vi "Validate Remote Session.vi"(0 "Session in":refnum<class "Remote Connection Session.lvclass">, 11 "error in":errorcluster) -> (4 "Session out":refnum<class "Remote Connection Session.lvclass">, 15 "error out":errorcluster)   [LabVIEW 2012, in "REx.lvlib" / "Remote Connection Session.lvclass"]
uses:
  Remote Connection Session.lvclass
  Remote Connection Session.lvclass/Remote Connection Session.ctl
  Local Listener Session/Obtain Session.vi
  Local Listener Session/Release Session.vi
  Local Listener Session/Local Listener Session.lvclass
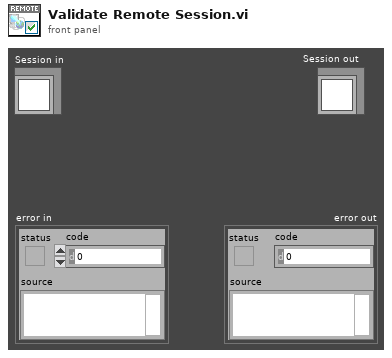
[diagram p1: front panel]
types:
  T1 = typedef "REx.lvlib/Local Listener Session.lvclass/Session Handle.ctl" = refnum<data-value>
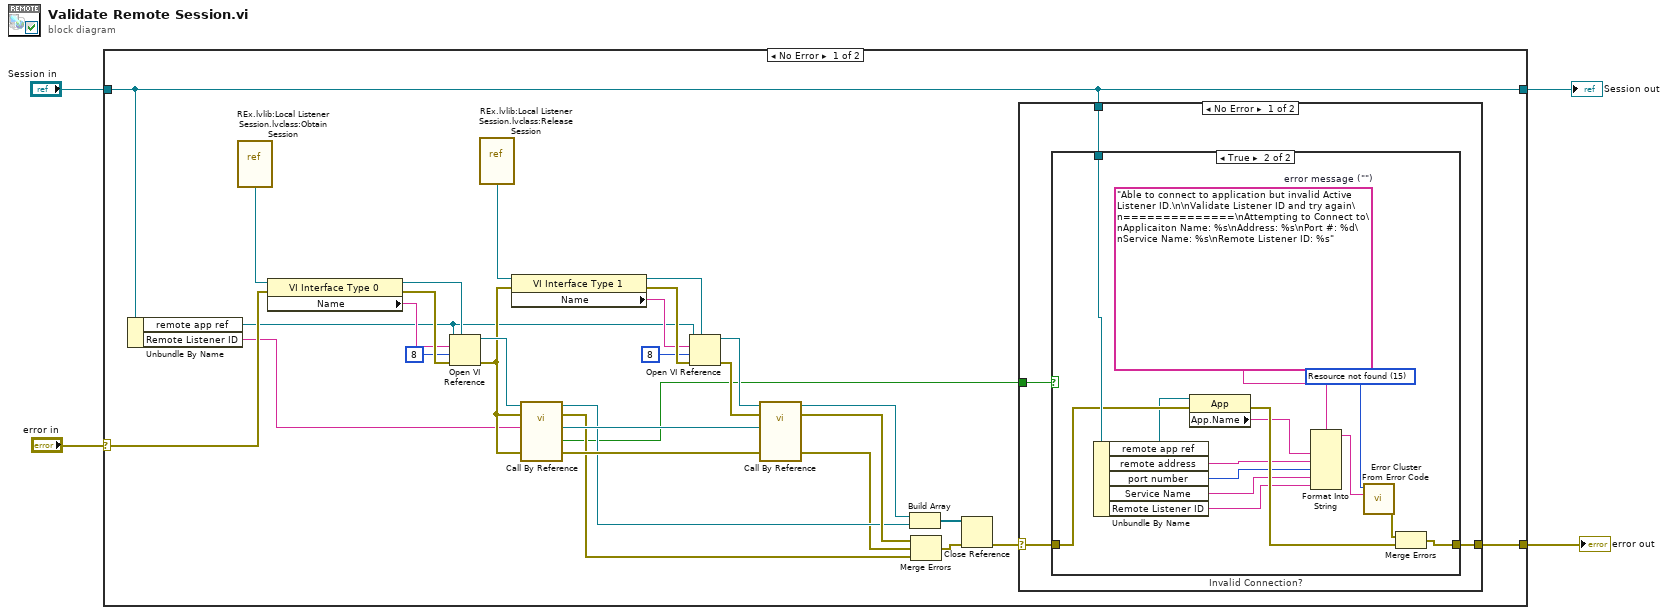
[diagram p0: block diagram]
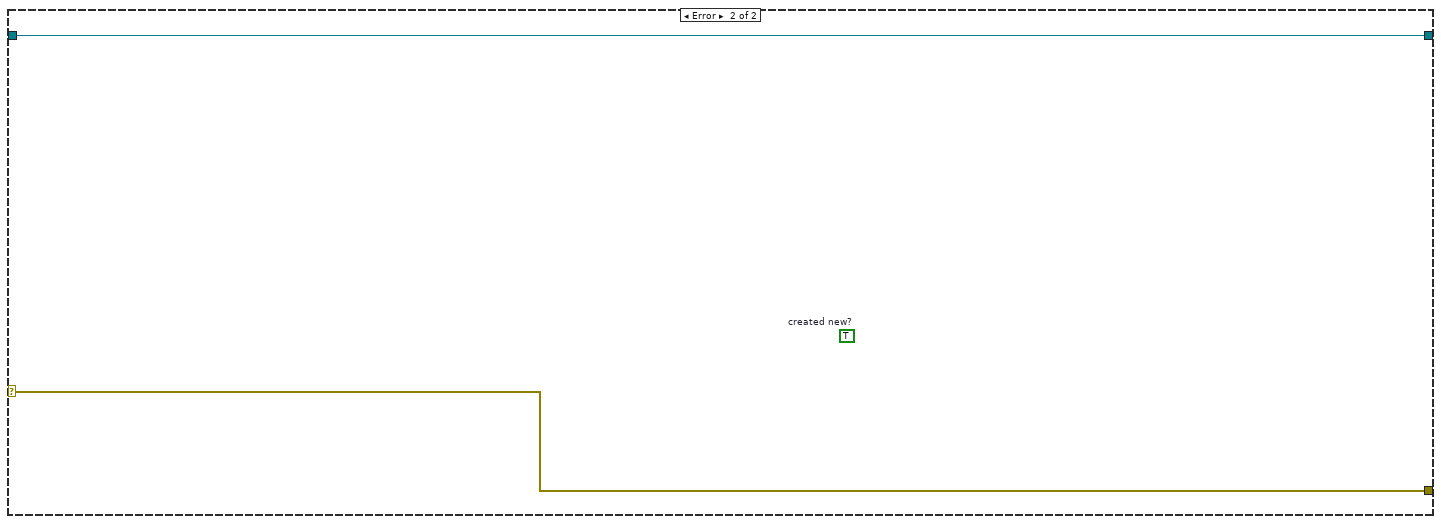
[diagram p4: hidden frame]
diagram:
  n1 = case shown="No Error" "error in" {
    selector: "error in" -> [w12 w55]
    tunnel: [w9 w55] -> w4
    tunnel: "Session in" -> [w7 w56]
    tunnel: [w7 w56] -> w1
    frame No Error {
      n2 = Unbundle By Name(w7) -> ("remote app ref"=w5:refnum<vi>, "Remote Listener ID"=w10:string)
      n3 = vi-ref "REx.lvlib:Local Listener Session.lvclass:Obtain Session.vi"() -> (w22:refnum<vi>)
      n4 = property class="VI Interface Type 0"(reference=w22, error in=w12) -> (reference out=w23:refnum<vi>, error out=w32:errorcluster, "Name"=w30:string)
      n5 = Open VI Reference(type specifier VI Refnum (for type only)=w23, application reference (local)=w5, vi path=w30, options=8, error in (no error)=w32) -> (vi reference=w29:refnum<vi>, error out=w11:errorcluster)  [unwired: 1 out]
      n6 = vi-ref "REx.lvlib:Local Listener Session.lvclass:Release Session.vi"() -> (w14:refnum<vi>)
      n7 = property class="VI Interface Type 1"(reference=w14, error in=w11) -> (reference out=w21:refnum<vi>, error out=w33:errorcluster, "Name"=w26:string)
      n8 = call-by-ref "?"(reference=w29, error in=w11, "Listener ID (REx Listener)"=w10, 11:"error in (no error)"=w11) -> (reference out=w19:refnum<vi>, error out=w17:errorcluster, "Listener Session Handle"=w24:T1, "created new?"=w6:bool, 15:"error out"=w20:errorcluster)  [unwired: 10 in, 1 out]
      n9 = Open VI Reference(type specifier VI Refnum (for type only)=w21, application reference (local)=w5, vi path=w26, options=8, error in (no error)=w33) -> (vi reference=w27:refnum<vi>, error out=w28:errorcluster)  [unwired: 1 out]
      n10 = call-by-ref "?"(reference=w27, error in=w28, "Session Handle"=w24, 11:"error in (no error)"=w20) -> (reference out=w15:refnum<vi>, error out=w34:errorcluster, 15:"error out"=w13:errorcluster)  [unwired: 13 in]
      n11 = Build Array(w15, w19) -> (w18:refnum<vi>[])
      n12 = Merge Errors(w34, w13, w17) -> (w16:errorcluster)
      n13 = Close Reference(reference=w18, error in (no error)=w16) -> (error out=w8:errorcluster)
      n14 = case shown="No Error" w8 {
        selector: w8 -> [w36 w54]
        tunnel: [w38 w54] -> w9
        tunnel: w7 -> [w37 _]
        tunnel: w6 -> [w35 _]
        frame No Error {
          n15 = case "Invalid Connection?" shown="True" w35 {
            tunnel: [w39 w52] -> w38
            tunnel: w37 -> [_ w51]
            tunnel: w36 -> [w39 w42]
            frame False {
            }
            frame True {
              w45 = 15 items=["No error", "Argument error", "Memory is full", "Out of zone", "End of file", "File already open", "Generic file I/O error", "File not found", "File permission error", "Disk is full", "Duplicate path", "Too many files open", "System feature not enabled", "Resource file not found", "Cannot add resource", "Resource not found", "Image not found", "Image memory error", "Pen does not exist", "Config type invalid", "Config token not found", "Config parse error", "Config memory error", "Bad external code format", "Bad external code offset", "External code not present", "Null window", "Destroy window error", "Null menu", "Print aborted", "Bad print record", "Print driver error", "Windows error during printing", "Memory error during printing", "Print dialog error", "Generic print error", "Invalid device refnum", "Device not found", "Device parameter error", "Device unit error", "Cannot open device", "Device call aborted", "Generic error", "Cancelled by user", "Object ID too low", "Object ID too high", "Object not in heap", "Unknown heap", "Unknown object (invalid DefProc)", "Unknown object (DefProc not in table)", "Message out of range", "Invalid (null) method", "Unknown message", "Manager call not supported", "Bad address", "Network operation in progress", "Network operation timed out", "Connection is busy", "Network attribute not supported", "Network error", "Address in use", "System out of memory", "Connection aborted", "Connection refused", "Not connected", "Already connected", "Connection closed", "Initialization error (interapplication manager)", "Bad occurrence", "Wait on unbound occurrence handler", "Occurrence queue overflow", "Datalog type conflict", "Unused", "Unrecognized type (interapplication manager)", "Memory corrupt", "Failed to make temporary DLL", "Old CIN version", "Drag socket not found", "Failed to load drop-object", "Failed to register OLE object", "Failed to release OLE object", "Format specifier type mismatch", "Unknown format specifier", "Too few format specifiers", "Too many format specifiers", "Scan failed", "Newer CIN version", "Error converting to variant", "Runtime menu error", "Password tampered", "Variant attribute not found", "Incompatible variant data type", "Event data is not available", "Event Store is not present", "Occurrence is not found", "Event Queue is not created", "Event info is not available", "Refnum passed is NULL", "Error retrieving Class GUID", "Error retrieving CoClass GUID", "Error retrieving TypeLib GUID.", "Bad built application magic bytes.", "Specific driver is different from the specific driver associated with the Logical Name.", "There is no session opened to the class driver.", "Max Error", "MAX - Error with config objects", "MAX - Error loading configuration", "MAX - Group not supported"]
              w46 = "Able to connect to application but invalid Active Listener ID.\n\nValidate Listener ID and try again\n==============\nAttempting to Connect to\nApplicaiton Name: %s\nAddress: %s\nPort #: %d\nService Name: %s\nRemote Listener ID: %s"  # error message ("")
              n16 = Unbundle By Name(w51) -> ("remote app ref"=w40:refnum<vi>, "remote address"=w50:string, "port number"=w49:u16, "Service Name"=w48:string, "Remote Listener ID"=w47:string)
              n17 = property class="App"(reference=w40, error in=w42) -> (error out=w53:errorcluster, "App.Name"=w41:string)  [unwired: 1 out]
              n18 = Format Into String(format string=w46, w41, w50, w49, w48, w47) -> (resulting string=w44:string)  [unwired: 2 in, 1 out]
              n19 = call <vilib>:"Error Cluster From Error Code.vi"("error message (\"\")"=w44, "error code (0)"=w45) -> ("error out"=w43:errorcluster)  [unwired: 7 in]
              n20 = Merge Errors(w43, w53) -> (w52:errorcluster)
            }
          }
        }
        frame Error {
        }
      }
    }
    frame Error {
      (unwired) TRUE  # created new?
    }
  }
  "error out" <- w4
  "Session out" <- w1
